vi "PSUN8731A-CTRLv31.vi"() -> ()   [LabVIEW 2017]
uses:
  Controller subVIs/CurrentPSUSettings.vi
  Keysight N8731A conversion/Keysight N8900 Series.lvlib
panel:
  out "Program ended":bool
  in  "Quench Protection":bool
  out "Status message":string
  out "TimeData":dbl[](array[numeric])
  out "VoltData":dbl[](array[numeric])
  out "CurrData":dbl[](array[numeric])
  out "StartTime":dbl
  out "I(t)":cluster{dbl[], dbl[]}(graph)
  out "V(t)":cluster{dbl[], dbl[]}(graph)
  in  "Sweep Controller":enum32{"Free Control Mode"}(tab)
  in  "Time between data points (ms)":i32=500 min=0
  out "Meas Voltage (V)":dbl
  out "Meas Current (A)":dbl
  in  "Voltage Set [V]":dbl min=0.0 max=8.0 step=0.001
  in  "Current Set [A]":dbl min=0.0 max=400.0 step=0.1
  in  "Power Output":bool
  in  "Voltmeter channel (6)":i32=6
  in  "End Program":bool
  out "Voltmeter error message":errorcluster
  in  "Voltmeter Range (V)":dbl caption="0 for Auto range"
  in  "Voltmeter Address (16)":i16=16
  out "PSU error message":errorcluster
  in  "OC protection":bool
  in  "OV Value (10V)":dbl=10.0 min=0.5 max=10.0
  out "I(V) Graph":cluster{dbl[], dbl[]}(graph)
  in  "VISA resource name":refnum<visa-resource-name>="N8731APSU"
  in  "Filename":string caption="Leave empty to discard data.\nDon't touch during measurement"
  in  "PSU\nVoltage":bool=TRUE caption="Keithley\nVoltage"
  in  "OV protection":bool=TRUE
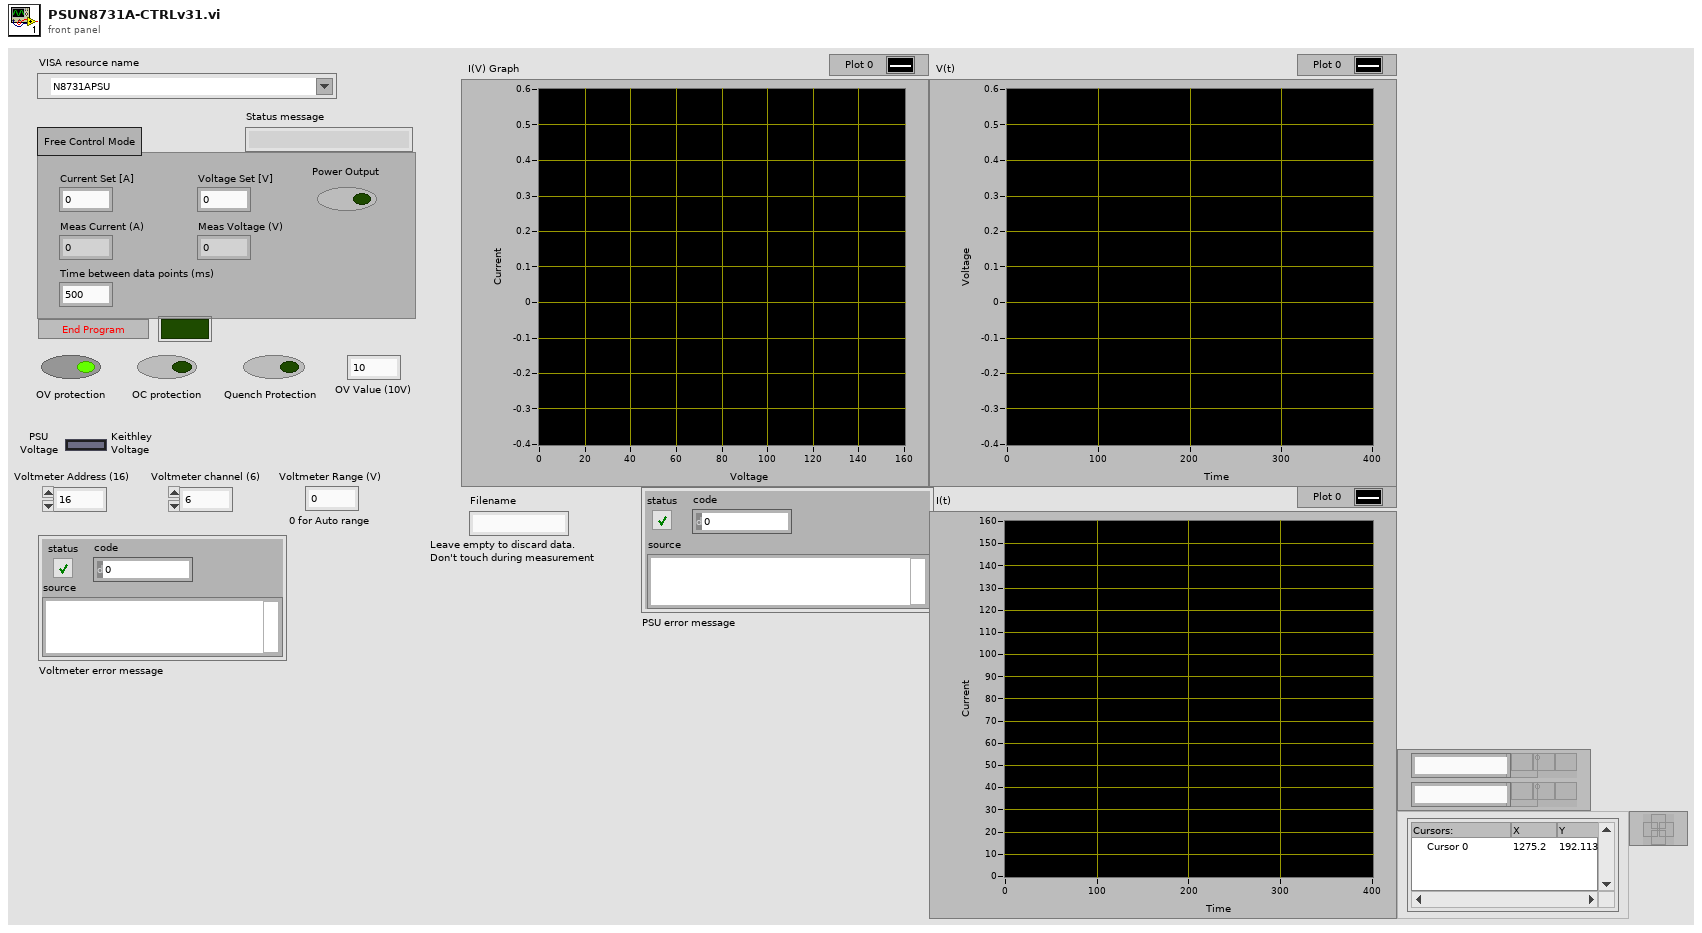
[diagram p1: front panel]
types:
  T1 = enum8{"Enabled", "Disabled", "Disabled and Grayed Out"}
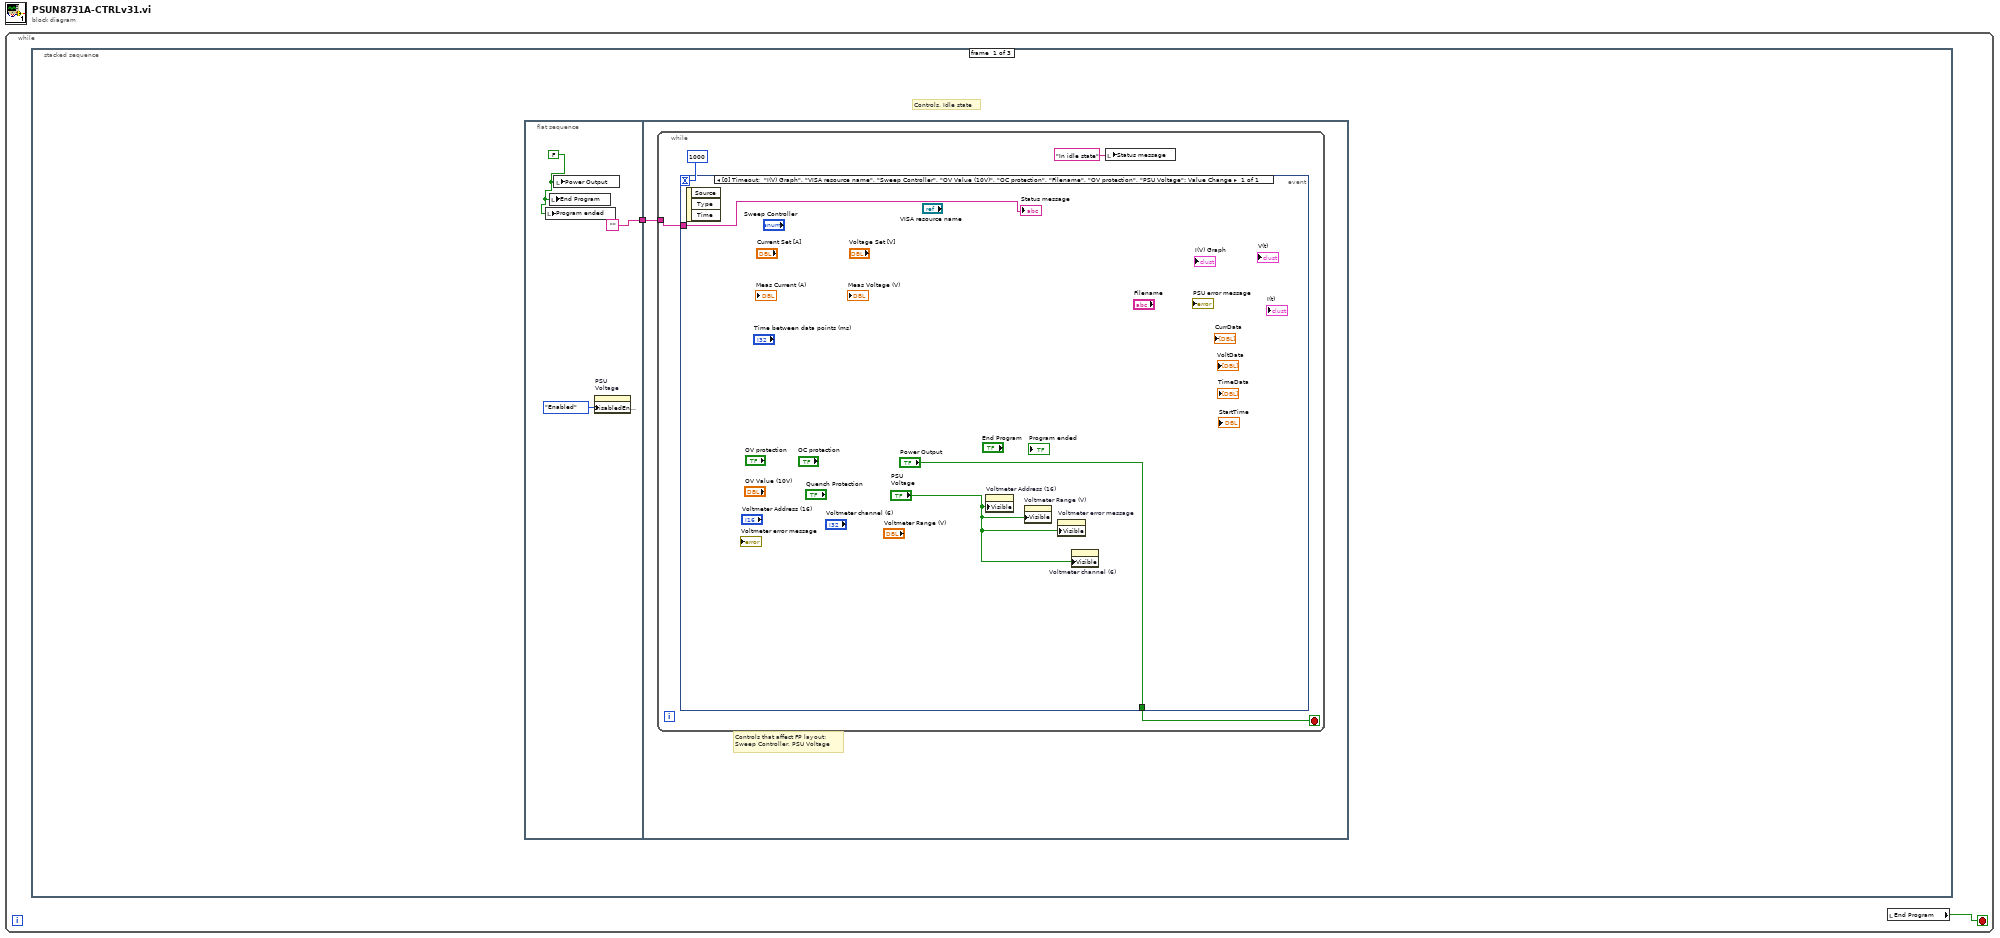
[diagram p0: block diagram]
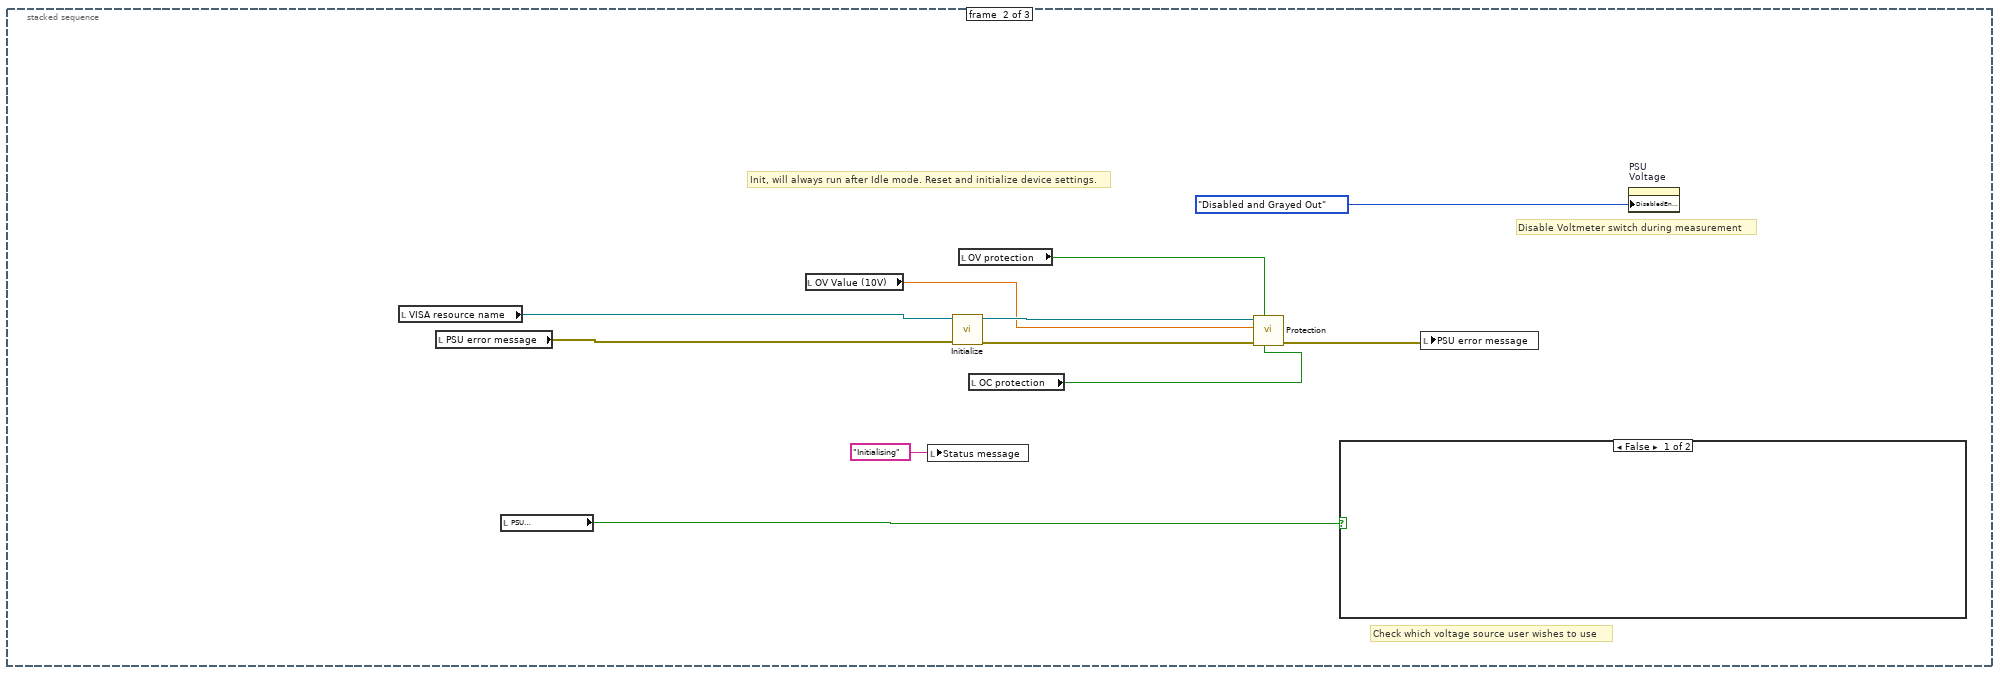
[diagram p2: hidden frame]
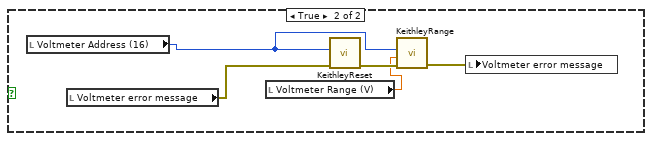
[diagram p3: hidden frame]
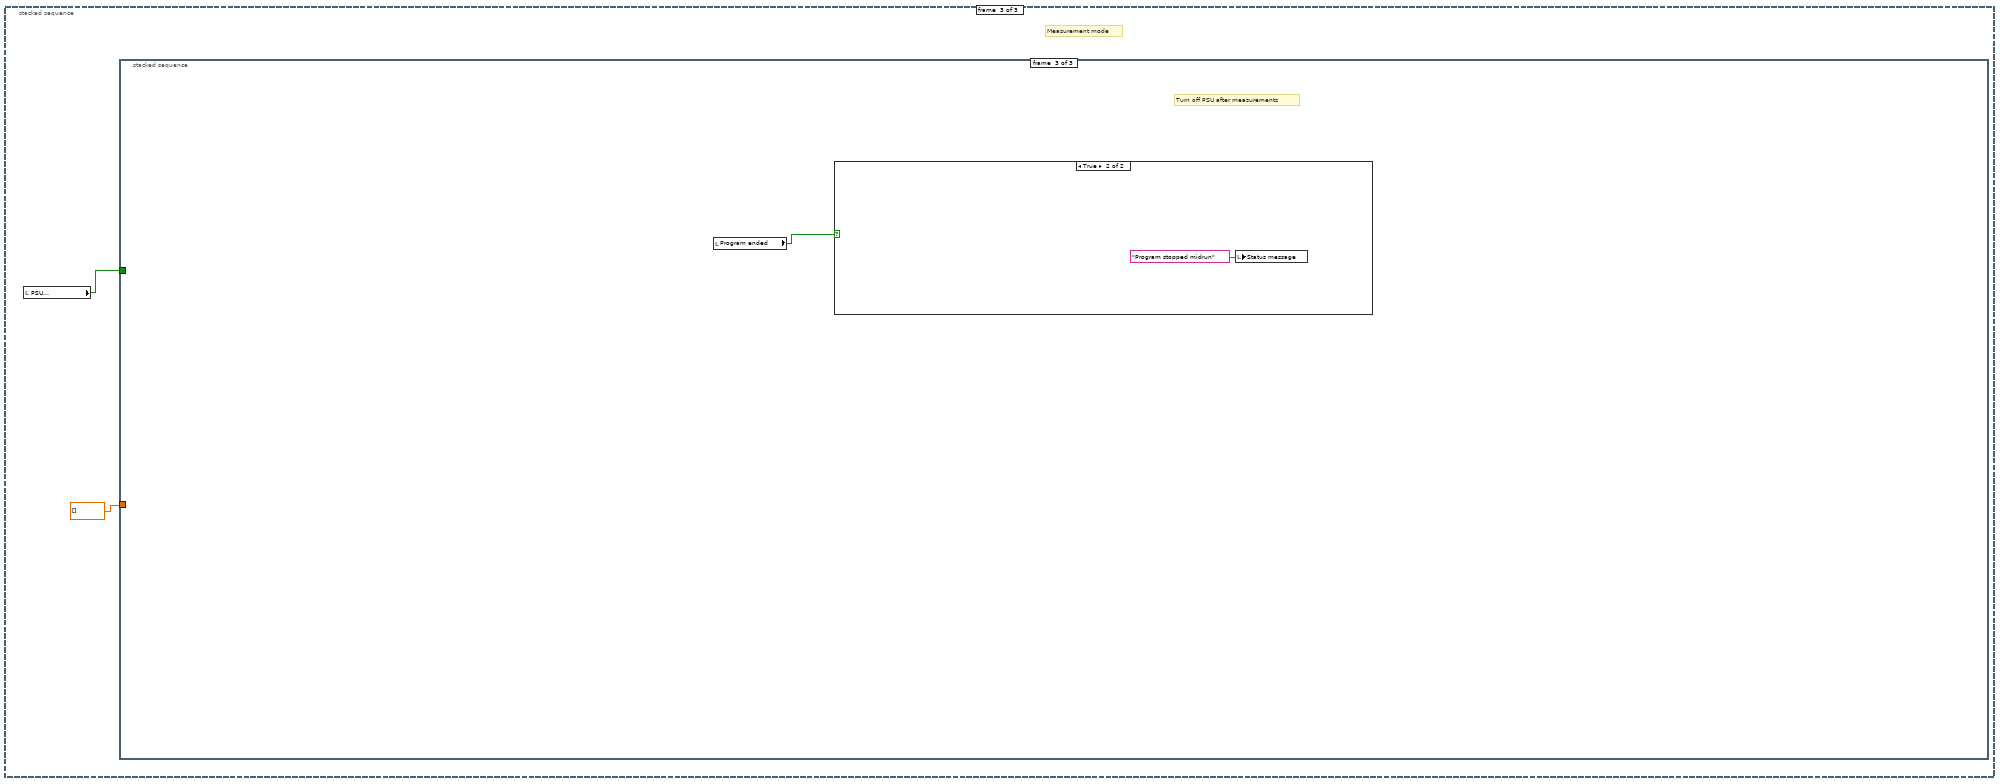
[diagram p4: hidden frame]
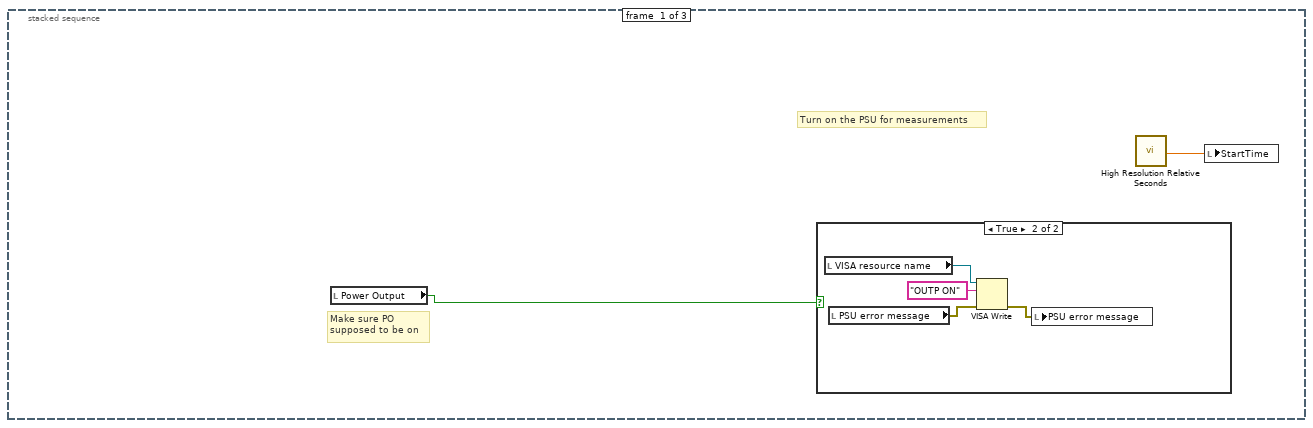
[diagram p5: hidden frame]
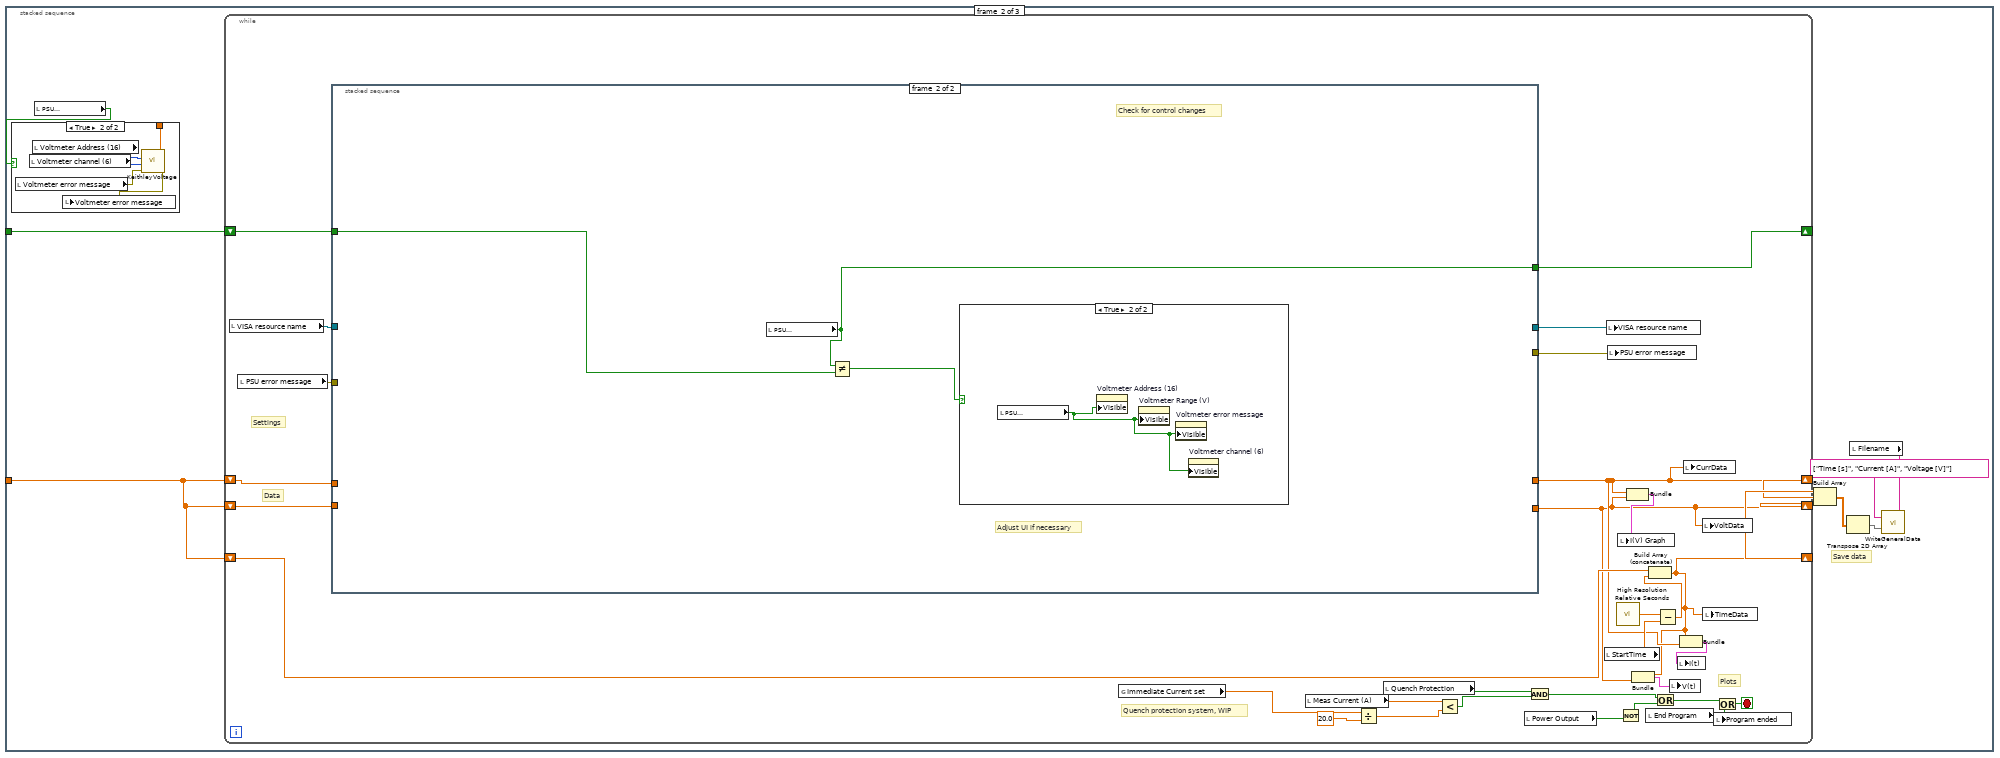
[diagram p7: hidden frame]
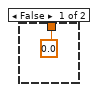
[diagram p8: hidden frame]
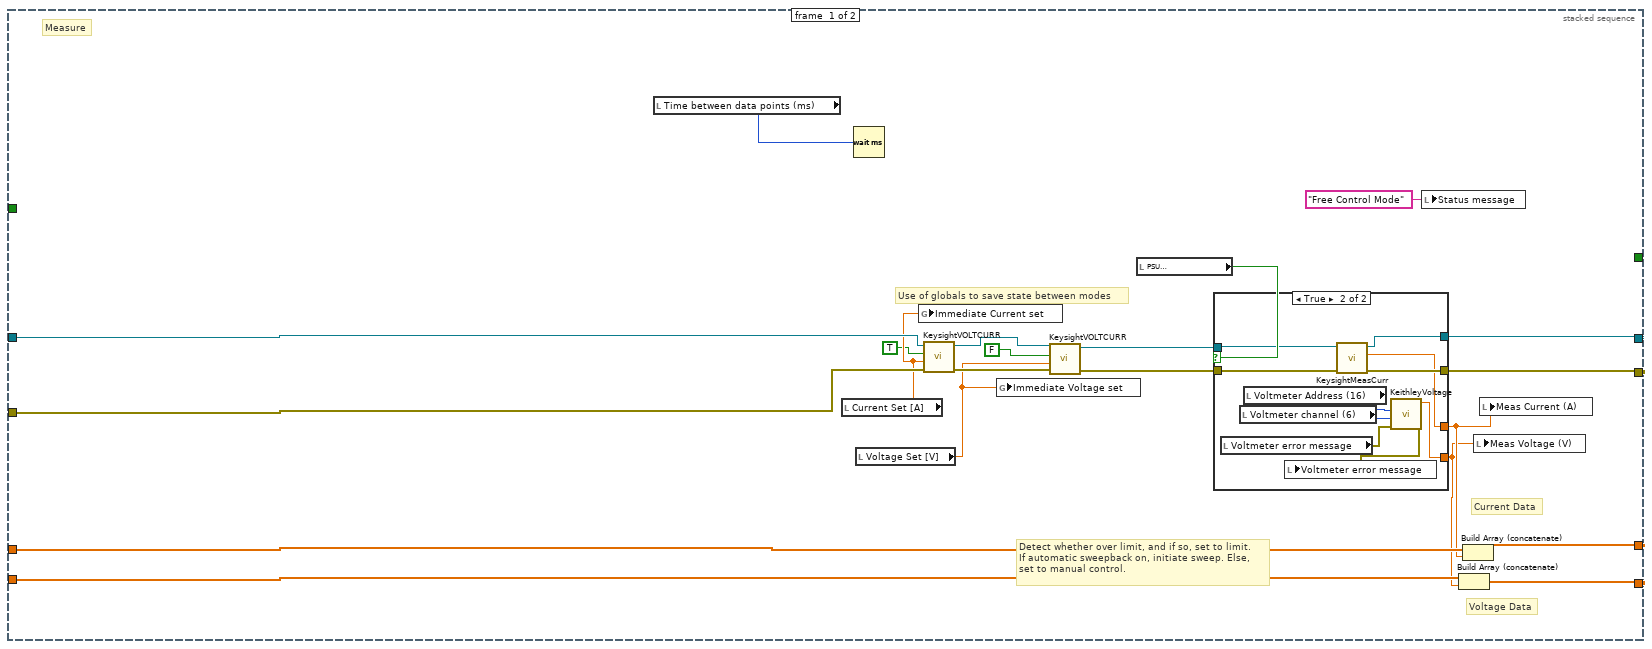
[diagram p9: hidden frame]
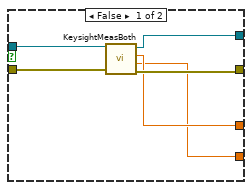
[diagram p10: hidden frame]
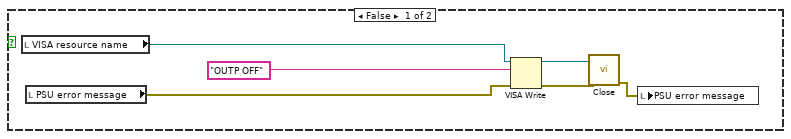
[diagram p12: hidden frame]
diagram:
  n1 = while {
    stop <- w1 stop-if-true
    n2 = stacked-sequence {
      frame #0 {
        # "Controls, Idle state"
        n3 = flat-sequence {
          tunnel: ["" ("Status message")] -> w2
          tunnel: w2 -> [w6]
          frame #0 {
            w3 = FALSE ("Sweeping Back")
            n4 = local write "Program ended"(w3) -> ()
            n5 = local write "End Program"(w3) -> ()
            n6 = local write "Power Output"(w3) -> ()
            n7 = property on="PSU\nVoltage" class="Bool (strict)"("DisabledEnum"=T1."Enabled" ("Disabled")) -> ()  [unwired: 2 in, 2 out]
          }
          frame #1 {
            # "Controls that affect FP layout:\nSweep Controller, PSU Voltage"
            n8 = while {
              tunnel: w6 -> [w8]
              stop <- w10 stop-if-true
              n9 = event shown="[0] Timeout;  \"I(V) Graph\", \"VISA resource name\", \"Sweep Controller\", \"OV Value (10V)\", \"OC protection\", \"Filename\", \"OV protection\", \"PSU Voltage\": Value Change" {
                selector: _ -> [_]
                dyn-events: _ -> [_]
                timeout: 1000 -> [_]
                tunnel: ["Power Output"] -> w10
                tunnel: w8 -> [w11]
                event Timeout; "I(V) Graph", "VISA resource name", "Sweep Controller", "OV Value (10V)", "OC protection", "Filename", "OV protection", "PSU\nVoltage": Value Change {
                  n10 = event-data() -> ()  [unwired: 1 in, 3 out]
                  n11 = property on="Voltmeter Address (16)" class="DigNum (strict)"("Visible"="PSU\nVoltage") -> ()  [unwired: 2 in, 2 out]
                  n12 = property on="Voltmeter Range (V)" class="DigNum (strict)"("Visible"="PSU\nVoltage") -> ()  [unwired: 2 in, 2 out]
                  n13 = property on="Voltmeter error message" class="Clust (strict)"("Visible"="PSU\nVoltage") -> ()  [unwired: 2 in, 2 out]
                  n14 = property on="Voltmeter channel (6)" class="DigNum (strict)"("Visible"="PSU\nVoltage") -> ()  [unwired: 2 in, 2 out]
                  "Status message" <- w11
                }
              }
              n15 = local write "Status message"("In idle state" ("Status message")) -> ()
            }
          }
        }
      }
      frame #1 {
        # "Check which voltage source user wishes to use"
        # "Disable Voltmeter switch during measurement"
        # "Init, will always run after Idle mode. Reset and initialize device settings."
        n16 = local read "VISA resource name"() -> (w22:refnum<visa-resource-name>)
        n17 = local read "PSU error message"() -> (w17:errorcluster)
        n18 = local read "PSU\nVoltage"() -> (w16:bool)
        n19 = local read "OV Value (10V)"() -> (w21:dbl)
        n20 = local write "Status message"("Initialising" ("Status message")) -> ()
        n21 = call "Initialize.vi"("error in (no error)"=w17, "VISA resource name"=w22) -> ("error out"=w23:errorcluster, "VISA resource name out"=w24:refnum<visa-resource-name>)  [unwired: 8 in]
        n22 = local read "OV protection"() -> (w19:bool)
        n23 = local read "OC protection"() -> (w20:bool)
        n24 = call "Protection.vi"("OC protection"=w20, "OV protection"=w19, "error in (no error)"=w23, "OV Value (10V)"=w21, "VISA resource name"=w24) -> ("error out"=w18:errorcluster)  [unwired: 5 in, 1 out]
        n25 = case shown="False" w16 {
          frame False {
          }
          frame True {
            n26 = local read "Voltmeter Address (16)"() -> (w25:i16)
            n27 = local read "Voltmeter error message"() -> (w27:errorcluster)
            n28 = local read "Voltmeter Range (V)"() -> (w26:dbl)
            n29 = call "KeithleyReset.vi"("error in"=w27, "address (16)"=w25) -> ("error out"=w28:errorcluster)  [unwired: 9 in]
            n30 = call "KeithleyRange.vi"("error in"=w28, "Range (V)/Auto(0)"=w26, "address (16)"=w25) -> ("error out"=w29:errorcluster)  [unwired: 8 in]
            n31 = local write "Voltmeter error message"(w29) -> ()
          }
        }
        n32 = local write "PSU error message"(w18) -> ()
        n33 = property on="PSU\nVoltage" class="Bool (strict)"("DisabledEnum"=T1."Disabled and Grayed Out" ("Disabled")) -> ()  [unwired: 2 in, 2 out]
      }
      frame #2 {
        # "Measurement mode"
        n34 = local read "PSU\nVoltage"() -> (w30:bool)
        n35 = stacked-sequence {
          tunnel: dbl[] [] -> [_ w47 _]
          tunnel: w30 -> [_ w38 _]
          frame #0 {
            # "Make sure PO\nsupposed to be on"
            # "Turn on the PSU for measurements"
            n36 = local read "Power Output"() -> (w33:bool)
            n37 = case shown="True" w33 {
              frame False {
              }
              frame True {
                n38 = local read "VISA resource name"() -> (w36:refnum<visa-resource-name>)
                n39 = local read "PSU error message"() -> (w35:errorcluster)
                n40 = VISA Write(VISA resource name=w36, write buffer="OUTP ON", error in (no error)=w35) -> (error out=w34:errorcluster)  [unwired: 2 out]
                n41 = local write "PSU error message"(w34) -> ()
              }
            }
            n42 = call <vilib>:"High Resolution Relative Seconds.vi"() -> ("relative seconds"=w32:dbl)
            n43 = local write "StartTime"(w32) -> ()
          }
          frame #1 {
            # "Save data"
            n44 = local read "PSU\nVoltage"() -> (w46:bool)
            n45 = case shown="True" w46 {
              tunnel: [0.0 ("Voltage") w49] -> _
              frame False {
              }
              frame True {
                n46 = local read "Voltmeter error message"() -> (w51:errorcluster)
                n47 = local read "Voltmeter channel (6)"() -> (w53:i32)
                n48 = local read "Voltmeter Address (16)"() -> (w52:i16)
                n49 = call "KeithleyVoltage.vi"("error in"=w51, "channel (6)"=w53, "address (16)"=w52) -> ("error out"=w50:errorcluster, "Voltage"=w49:dbl)  [unwired: 7 in]
                n50 = local write "Voltmeter error message"(w50) -> ()
              }
            }
            n51 = while {
              shift-right: [w57] -> _
              shift-left: w38 -> [w58]
              shift-right: [w62] -> w42
              shift-left: w47 -> [w79]
              shift-right: [w61] -> w41
              shift-left: w47 -> [w78]
              shift-right: [w60] -> w43
              shift-left: w47 -> [w75]
              stop <- w55 stop-if-true
              # "Plots"
              # "Quench protection system, WIP"
              # "Data"
              # "Settings"
              n52 = local read "VISA resource name"() -> (w83:refnum<visa-resource-name>)
              n53 = local read "PSU error message"() -> (w82:errorcluster)
              n54 = stacked-sequence {
                tunnel: w83 -> [w104 _]
                tunnel: w82 -> [w103 _]
                tunnel: [w102 _] -> w81
                tunnel: [w101 _] -> w80
                tunnel: w79 -> [w100 _]
                tunnel: [w99 _] -> w62
                tunnel: w78 -> [w98 _]
                tunnel: [w97 _] -> w61
                tunnel: w58 -> [_ w122]
                tunnel: [_ w121] -> w57
                frame #0 {
                  # "Use of globals to save state between modes"
                  # "Detect whether over limit, and if so, set to limit.\nIf automatic sweepback on, initiate sweep. Else,\nset to manual control."
                  # "Voltage Data"
                  # "Current Data"
                  # "Measure"
                  n55 = local read "Time between data points (ms)"() -> (w85:i32)
                  n56 = local read "Current Set [A]"() -> (w96:dbl)
                  n57 = Wait (ms)(milliseconds to wait=w85) -> ()  [unwired: 1 out]
                  n58 = local read "Voltage Set [V]"() -> (w87:dbl)
                  n59 = global write "CurrentPSUSettings.vi" "Immediate Current set"(w96) -> ()
                  n60 = call "KeysightVOLTCURR.vi"("error in (no error)"=w103, "CURR/VOLT (A/V)"=w96, "CURR (1)/VOLT (0)"=TRUE, "VISA resource name"=w104) -> ("error out"=w92:errorcluster, "VISA resource name out"=w93:refnum<visa-resource-name>)  [unwired: 6 in]
                  n61 = global write "CurrentPSUSettings.vi" "Immediate Voltage set"(w87) -> ()
                  n62 = call "KeysightVOLTCURR.vi"("error in (no error)"=w92, "CURR/VOLT (A/V)"=w87, "CURR (1)/VOLT (0)"=FALSE, "VISA resource name"=w93) -> ("error out"=w89:errorcluster, "VISA resource name out"=w90:refnum<visa-resource-name>)  [unwired: 6 in]
                  n63 = local read "PSU\nVoltage"() -> (w91:bool)
                  n64 = case shown="True" w91 {
                    tunnel: w90 -> [w110 w120]
                    tunnel: w89 -> [w109 w119]
                    tunnel: [w108 w114] -> w102
                    tunnel: [w107 w113] -> w101
                    tunnel: [w106 w112] -> w88
                    tunnel: [w105 w111] -> w86
                    frame False {
                      n65 = call "KeysightMeasBoth.vi"("error in (no error)"=w109, "VISA resource name"=w110) -> ("error out"=w107:errorcluster, "VOLT"=w105:dbl, "CURR"=w106:dbl, "VISA resource name out"=w108:refnum<visa-resource-name>)  [unwired: 6 in]
                    }
                    frame True {
                      n66 = local read "Voltmeter error message"() -> (w116:errorcluster)
                      n67 = local read "Voltmeter channel (6)"() -> (w118:i32)
                      n68 = local read "Voltmeter Address (16)"() -> (w117:i16)
                      n69 = call "KeysightMeasCurr.vi"("error in (no error)"=w119, "VISA resource name"=w120) -> ("error out"=w113:errorcluster, "CURR"=w112:dbl, "VISA resource name out"=w114:refnum<visa-resource-name>)  [unwired: 7 in]
                      n70 = call "KeithleyVoltage.vi"("error in"=w116, "channel (6)"=w118, "address (16)"=w117) -> ("error out"=w115:errorcluster, "Voltage"=w111:dbl)  [unwired: 7 in]
                      n71 = local write "Voltmeter error message"(w115) -> ()
                    }
                  }
                  n72 = local write "Status message"("Free Control Mode" ("Status message")) -> ()
                  n73 = Build Array (concatenate)(w98, w86) -> (w97:dbl[])
                  n74 = Build Array (concatenate)(w100, w88) -> (w99:dbl[])
                  n75 = local write "Meas Voltage (V)"(w86) -> ()
                  n76 = local write "Meas Current (A)"(w88) -> ()
                }
                frame #1 {
                  # "Adjust UI if necessary"
                  # "Check for control changes"
                  n77 = local read "PSU\nVoltage"() -> (w121:bool)
                  n78 = Not Equal?(x=w121, y=w122) -> (x != y?=w123:bool)
                  n79 = case shown="True" w123 {
                    frame False {
                    }
                    frame True {
                      n80 = local read "PSU\nVoltage"() -> (w124:bool)
                      n81 = property on="Voltmeter Address (16)" class="DigNum (strict)"("Visible"=w124) -> ()  [unwired: 2 in, 2 out]
                      n82 = property on="Voltmeter Range (V)" class="DigNum (strict)"("Visible"=w124) -> ()  [unwired: 2 in, 2 out]
                      n83 = property on="Voltmeter error message" class="Clust (strict)"("Visible"=w124) -> ()  [unwired: 2 in, 2 out]
                      n84 = property on="Voltmeter channel (6)" class="DigNum (strict)"("Visible"=w124) -> ()  [unwired: 2 in, 2 out]
                    }
                  }
                }
              }
              n85 = global read "CurrentPSUSettings.vi" "Immediate Current set"() -> (w67:dbl)
              n86 = local read "Meas Current (A)"() -> (w68:dbl)
              n87 = Divide(x=w67, y=20.0) -> (x/y=w65:dbl)
              n88 = local read "Quench Protection"() -> (w59:bool)
              n89 = Less?(x=w68, y=w65) -> (x < y?=w69:bool)
              n90 = local read "Power Output"() -> (w76:bool)
              n91 = And(x=w59, y=w69) -> (x .and. y?=w63:bool)
              n92 = local read "StartTime"() -> (w73:dbl)
              n93 = local write "VISA resource name"(w81) -> ()
              n94 = local write "PSU error message"(w80) -> ()
              n95 = call <vilib>:"High Resolution Relative Seconds.vi"() -> ("relative seconds"=w74:dbl)
              n96 = Not(x=w76) -> (.not. x?=w64:bool)
              n97 = Bundle(w62, w61) -> (w77:cluster{dbl[], dbl[]})  [unwired: 1 in]
              n98 = local write "I(V) Graph"(w77) -> ()
              n99 = local read "End Program"() -> (w54:bool)
              n100 = Or(x=w63, y=w64) -> (x .or. y?=w56:bool)
              n101 = Subtract(x=w74, y=w73) -> (x-y=w72:dbl)
              n102 = Build Array (concatenate)(w75, w72) -> (w60:dbl[])
              n103 = Bundle(w60, w61) -> (w71:cluster{dbl[], dbl[]})  [unwired: 1 in]
              n104 = local write "V(t)"(w71) -> ()
              n105 = Bundle(w60, w62) -> (w70:cluster{dbl[], dbl[]})  [unwired: 1 in]
              n106 = local write "I(t)"(w70) -> ()
              n107 = local write "CurrData"(w62) -> ()
              n108 = local write "VoltData"(w61) -> ()
              n109 = local write "TimeData"(w60) -> ()
              n110 = local write "Program ended"(w54) -> ()
              n111 = Or(x=w56, y=w54) -> (x .or. y?=w55:bool)
            }
            n112 = Build Array(w43, w42, w41) -> (w39:dbl[][])
            n113 = Transpose 2D Array(2D array=w39) -> (transposed array=w40:dbl[][])
            n114 = local read "Filename"() -> (w45:string)
            n115 = call "WriteGeneralData.vi"("filename (discard if empty)"=w45, "Array"=w40, "Column name array"=string[] ["Time [s]", "Current [A]", "Voltage [V]"]) -> ()
          }
          frame #2 {
            # "Turn off PSU after measurements"
            n116 = local read "Program ended"() -> (w125:bool)
            n117 = case shown="True" w125 {
              frame False {
                n118 = local read "VISA resource name"() -> (w131:refnum<visa-resource-name>)
                n119 = local read "PSU error message"() -> (w130:errorcluster)
                n120 = VISA Write(VISA resource name=w131, write buffer="OUTP OFF", error in (no error)=w130) -> (VISA resource name out=w128:refnum<visa-resource-name>, error out=w127:errorcluster)  [unwired: 1 out]
                n121 = call "Close.vi"("error in (no error)"=w127, "VISA resource name"=w128) -> ("error out"=w126:errorcluster)  [unwired: 9 in]
                n122 = local write "PSU error message"(w126) -> ()
              }
              frame True {
                n123 = local write "Status message"("Program stopped midrun" ("Status message")) -> ()
              }
            }
          }
        }
      }
    }
    n124 = local read "End Program"() -> (w1:bool)
  }
